vi "Initialize.vi"(7 "Process ID":string, 8 "error in (no error)":errorcluster, 11 "Assembler in":refnum<class "Assembler.lvclass">) -> (0 "error out":errorcluster, 3 "Assembler out":refnum<class "Assembler.lvclass">)   [LabVIEW 2019, in "TimingDRV Engine.lvlib" / "Assembler.lvclass"]
uses:
  Assembler.lvclass
  C:/Users/XEnderMD/Desktop/CD Project Tools/Source/Engine/Parent Classes/Process/Process.lvclass
  Assembler.lvclass/Assembler.ctl
  Parent Classes/Process/Process.lvclass/Process.ctl
  Parent Classes/Process/Accessors/Process ID/Get Process ID.vi
  Parent Classes/Process/Accessors/Process UEs/Set Process UEs.vi
  Parent Classes/Process/Accessors/Process Qs/Set Process Qs.vi
  Parent Classes/Process/Accessors/Process IDs/Set Process IDs.vi
  Parent Classes/Process/Process.lvclass
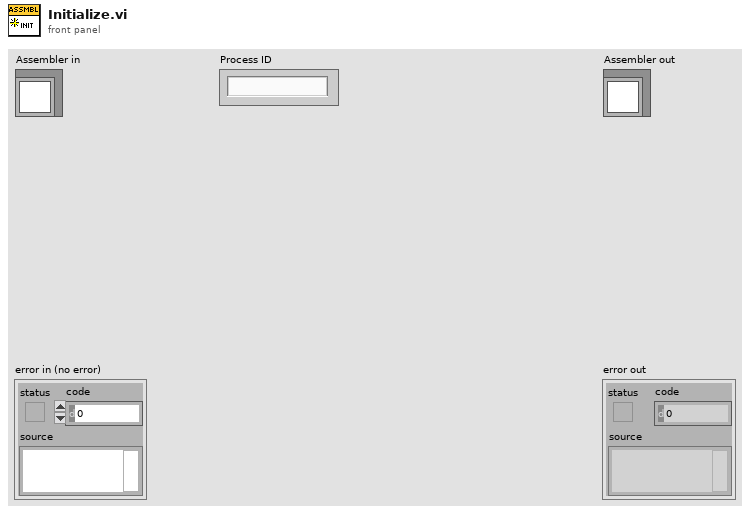
[diagram p1: front panel]
types:
  T1 = typedef "TimingDRV Engine.lvlib/Process.lvclass/Process Lookup.ctl" = cluster{"Process ID":string, "MessageQ":refnum<queue>, "Update UE":refnum<user-event>}
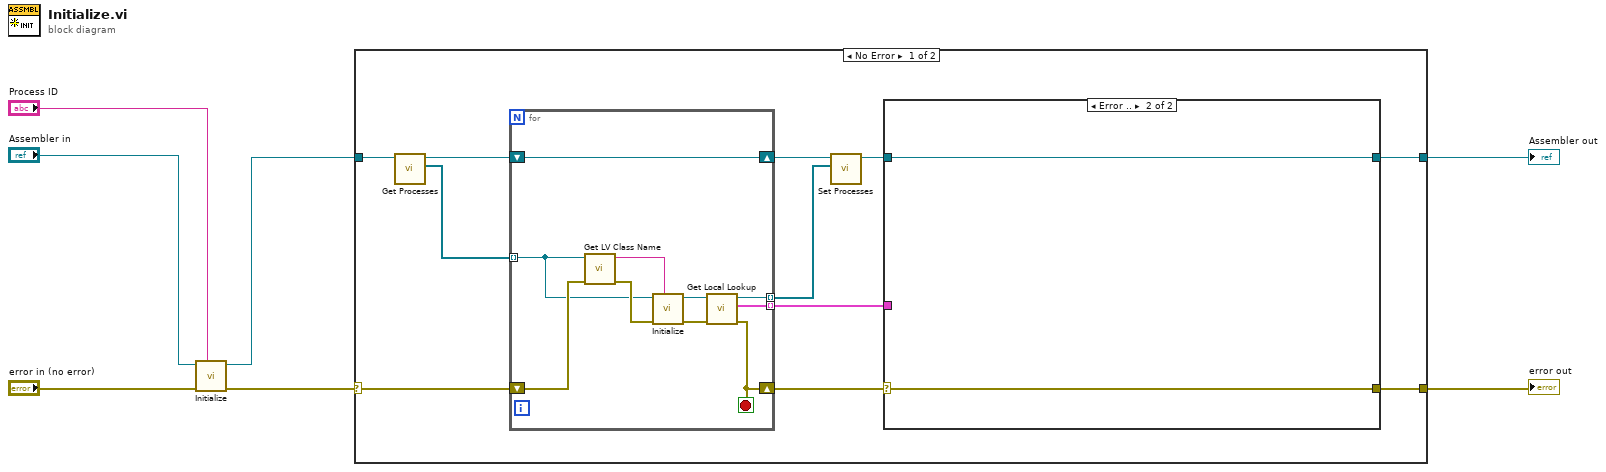
[diagram p0: block diagram]
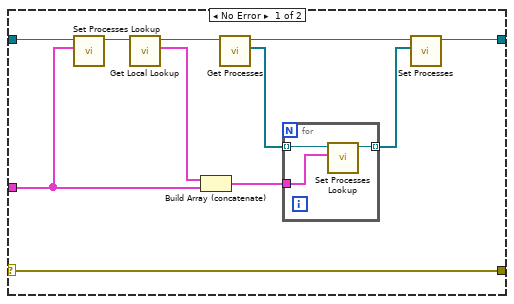
[diagram p2: hidden frame]
diagram:
  n1 = call-parent "Initialize.vi"("Process ID"="Process ID", "error in (no error)"="error in (no error)", "Process in"="Assembler in") -> ("error out"=w2:errorcluster, "Process out"=w3:refnum<class "Assembler.lvclass">)  [unwired: 7 in]
  n2 = case shown="No Error" w2 {
    selector: w2 -> [w18 w45]
    tunnel: w3 -> [w8 w46]
    tunnel: [w12 w46] -> w4
    tunnel: [w11 w45] -> w1
    frame No Error {
      n3 = call "Get Processes.vi"("Assembler in"=w8) -> ("Processes"=w10:refnum<class "Process.lvclass">[], "Assembler out"=w9:refnum<class "Assembler.lvclass">)  [unwired: 9 in]
      n4 = for {
        tunnel: w10 -> [w41] mode=indexing
        shift-right: [w40] -> w17
        shift-left: w9 -> [w40]
        shift-right: [w36] -> w14
        shift-left: w18 -> [w42]
        tunnel: [w38] -> w16 mode=indexing
        tunnel: [w35] -> w13 mode=indexing
        stop <- w36 stop-if-true
        n5 = call <vilib>:"Get LV Class Name.vi"("error in (no error)"=w42, "object"=w41) -> ("error out"=w44:errorcluster, "class name"=w43:string)  [unwired: 8 in]
        n6 = call-dynamic "Initialize.vi"("Process ID"=w43, "error in (no error)"=w44, "Process in"=w41) -> ("error out"=w37:errorcluster, "Process out"=w39:refnum<class "Process.lvclass">)  [unwired: 7 in]
        n7 = call-dynamic "Get Local Lookup.vi"("error in (no error)"=w37, "Process in"=w39) -> ("error out"=w36:errorcluster, "Process Lookup"=w35:T1, "Process out"=w38:refnum<class "Process.lvclass">)  [unwired: 7 in]
      }
      n8 = call "Set Processes.vi"("Processes"=w16, "Assembler in"=w17) -> ("Assembler out"=w15:refnum<class "Assembler.lvclass">)  [unwired: 9 in]
      n9 = case shown="Error .." w14 {
        selector: w14 -> [w22 w33]
        tunnel: w15 -> [w21 w34]
        tunnel: w13 -> [w19 _]
        tunnel: [w23 w34] -> w12
        tunnel: [w22 w33] -> w11
        frame No Error {
          n10 = call "Set Processes Lookup.vi"("Processes Lookup"=w19, "Process in"=w21) -> ("Process out"=w20:refnum<class "Assembler.lvclass">)  [unwired: 9 in]
          n11 = call-dynamic "Get Local Lookup.vi"("Process in"=w20) -> ("Process Lookup"=w26:T1, "Process out"=w27:refnum<class "Assembler.lvclass">)  [unwired: 8 in, 1 out]
          n12 = Build Array (concatenate)(w26, w19) -> (w25:T1[])
          n13 = call "Get Processes.vi"("Assembler in"=w27) -> ("Processes"=w29:refnum<class "Process.lvclass">[], "Assembler out"=w28:refnum<class "Assembler.lvclass">)  [unwired: 9 in]
          n14 = for {
            tunnel: w29 -> [w32] mode=indexing
            tunnel: w25 -> [w31]
            tunnel: [w30] -> w24 mode=indexing
            n15 = call "Set Processes Lookup.vi"("Processes Lookup"=w31, "Process in"=w32) -> ("Process out"=w30:refnum<class "Process.lvclass">)  [unwired: 9 in]
          }
          n16 = call "Set Processes.vi"("Processes"=w24, "Assembler in"=w28) -> ("Assembler out"=w23:refnum<class "Assembler.lvclass">)  [unwired: 9 in]
        }
        frame Error {
        }
      }
    }
    frame Error {
    }
  }
  "error out" <- w1
  "Assembler out" <- w4
